vi "From String Array.vi"(8 "error in (no error)":errorcluster, 9 "String Array":string[](array[string]), 11 "String Compare Config in":refnum<class "String Compare Config.lvclass">) -> (0 "error out":errorcluster, 1 "String Array 2":string[](array[string]), 2 "Version":string, 3 "String Compare Config out":refnum<class "String Compare Config.lvclass">)   [LabVIEW 2015, in "String Compare Config.lvclass"]
uses:
  String Compare Config.lvclass
  <vilib>/NI/Tag Bus/tag/Data Type.ctl
  <vilib>/NI/Tag Bus Module Framework/channel/channel classification.ctl
  Mode.ctl
  String Compare Config.lvclass/String Compare Config.ctl
  Write Test Value Channel.vi
  Write Result Channel.vi
  Write Mode.vi
  Write Limit_Regex.vi
  Write ignore case.vi
  Write Multiline.vi
  Write offset.vi
  classes/Step/Config/Step Config.lvclass
  <vilib>/NI/Tag Bus Module Framework/channel/TBM channel.lvclass
  <vilib>/NI/Tag Bus/tag/tag descriptor.lvclass
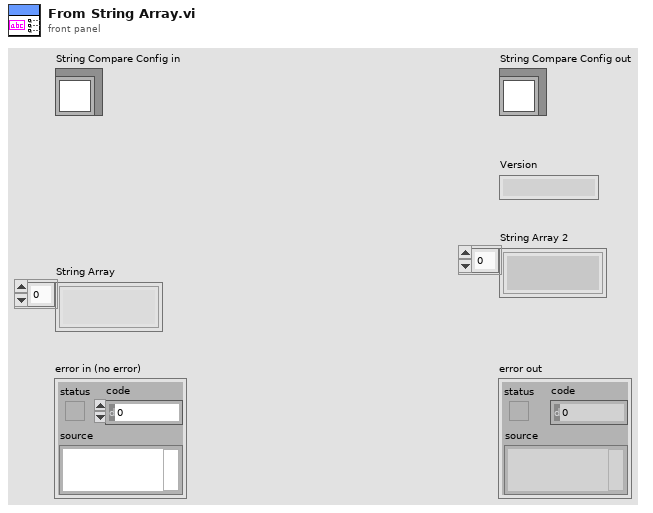
[diagram p1: front panel]
types:
  T1 = typedef "TBM channel.lvclass/channel classification.ctl" = enum16{"input data", "output data", "processing parameter", "processing result"}
  T2 = typedef "tag bus.lvlib/tag descriptor.lvclass/Data Type.ctl" = enum16{"Double", "Single", "I64", "I32", "I16", "I8", "U64", "U32", "U16", "U8", "Boolean", "String", "Array of Double", "Array of Single", "Array of I64", "Array of I32", "Array of I16", "Array of I8", "Array of U64", "Array of U32", "Array of U16", "Array of U8", "Array of Boolean", "Array of String"}
  T3 = typedef "String Compare Config.lvclass/Mode.ctl" = enum16{"Compare Strings", "Match Regex"}
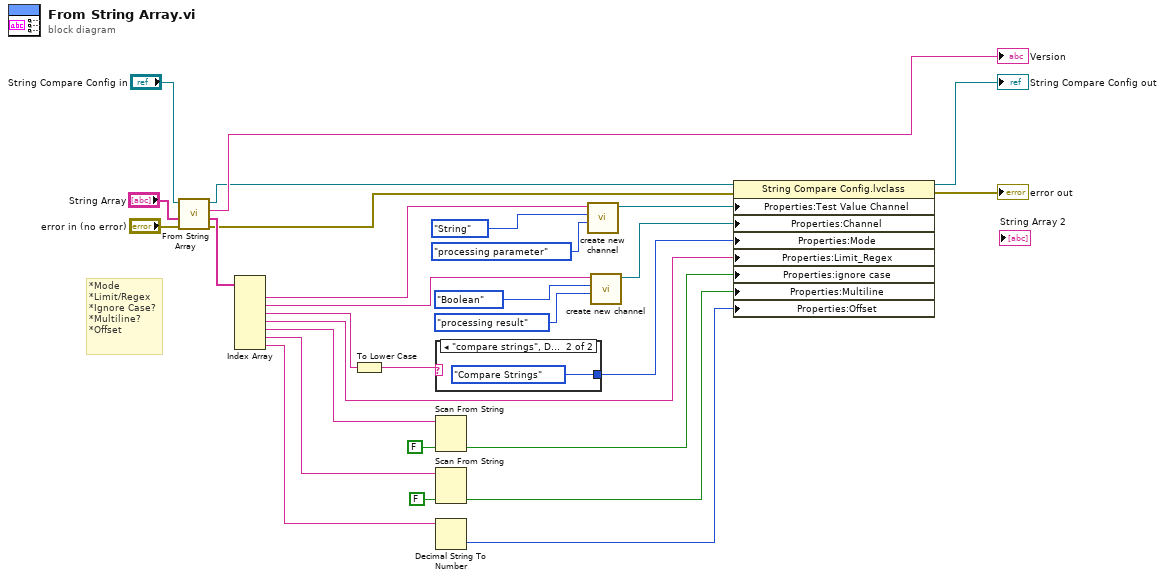
[diagram p0: block diagram]
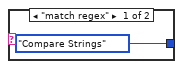
[diagram p2: hidden frame]
diagram:
  # "*Mode\n*Limit/Regex\n*Ignore Case?\n*Multiline?\n*Offset"
  n1 = call-parent "From String Array.vi"("error in (no error)"="error in (no error)", "String Array"="String Array", "Step Config in"="String Compare Config in") -> ("error out"=w23:errorcluster, "Elements Left"=w25:string[], "Version"=→"Version":string, "Step Config out"=w24:refnum<class "String Compare Config.lvclass">)  [unwired: 5 in]
  n2 = Index Array(array=w25) -> (element #1=w2:string, element #2=w1:string, element #3=w3:string, element #4=w4:string, element #5=w5:string, element #6=w6:string, element #7=w7:string)  [unwired: 7 in]
  n3 = To Lower Case(string=w3) -> (all lower case string=w15:string)
  n4 = case shown="\"compare strings\", Default" w15 {
    tunnel: [Mode."Compare Strings" ("Mode") Mode."Compare Strings" ("Mode")] -> w14
    frame "match regex" {
    }
    frame "compare strings", Default {
    }
  }
  n5 = Scan From String(input string=w5, default 1=FALSE ("Negate Result")) -> (output 1=w12:bool)  [unwired: 3 in, 3 out]
  n6 = Scan From String(input string=w6, default 1=FALSE ("Negate Result")) -> (output 1=w10:bool)  [unwired: 3 in, 3 out]
  n7 = Decimal String To Number(string=w7) -> (number=w9:i32)  [unwired: 2 in, 1 out]
  n8 = call <vilib>:"create new channel.vi"("channel classification"=channel_classification."processing parameter", "data type"=Data_Type."String", "channel name"=w2) -> ("channel"=w17:refnum<class "TBM channel.lvclass">)  [unwired: 8 in]
  n9 = call <vilib>:"create new channel.vi"("channel classification"=channel_classification."processing result", "data type"=Data_Type."Boolean", "channel name"=w1) -> ("channel"=w16:refnum<class "TBM channel.lvclass">)  [unwired: 8 in]
  n10 = property class="String Compare Config.lvclass"(reference=w24, error in=w23, "Properties:Test Value Channel"=w17, "Properties:Channel"=w16, "Properties:Mode"=w14, "Properties:Limit_Regex"=w4, "Properties:ignore case"=w12, "Properties:Multiline"=w10, "Properties:Offset"=w9) -> (reference out=→"String Compare Config out":refnum<class "String Compare Config.lvclass">, error out=→"error out":errorcluster)
